vi "题目5.vi"() -> ()   [LabVIEW 2017]
panel:
  out "恭喜":bool
  out "?":bool
  out "警告":bool
  in  "数值":dbl
  # "通过"
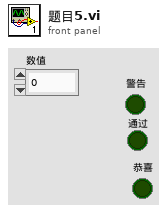
[diagram p1: front panel]
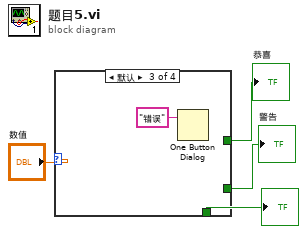
[diagram p0: block diagram]
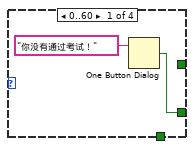
[diagram p2: hidden frame]
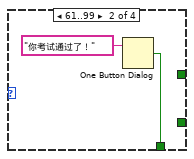
[diagram p3: hidden frame]
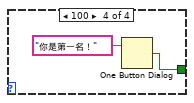
[diagram p4: hidden frame]
diagram:
  n1 = case shown="默认" "数值" {
    tunnel: [_ _ _ w10] -> w3
    tunnel: [w5 _ _ _] -> w2
    tunnel: [_ w7 _ _] -> w1
    frame 0..60 {
      n2 = One Button Dialog(message="你没有通过考试！" ("消息")) -> (true=w5:bool)  [unwired: 1 in]
    }
    frame 61..99 {
      n3 = One Button Dialog(message="你考试通过了！" ("消息")) -> (true=w7:bool)  [unwired: 1 in]
    }
    frame Default {
      n4 = One Button Dialog(message="错误" ("消息")) -> ()  [unwired: 1 in, 1 out]
    }
    frame 100 {
      n5 = One Button Dialog(message="你是第一名！" ("消息")) -> (true=w10:bool)  [unwired: 1 in]
    }
  }
  "恭喜" <- w3
  "警告" <- w2
  "?" <- w1
